vi "IMAG32at.VI"() -> ()   [LabVIEW 2013]
uses:
  Program Files/Andor SOLIS/Drivers 32bit/Examples/LabVIEW/System Files/user.lib/atmcd32d.llb/Shutter_type typedef.ctl
panel:
  out "Intensity Graph":i32[][](graph)
  out "Detector Y Pixels":i32
  in  "Shutter Trigger":T1
  in  "Time to open or\nclose shutter (ms):":i32=50
  in  "Shut Down":bool
  in  "Start Acquisition":bool
  out "Return  from Get Acquired Data":u32
  out "Detector X Pixels":i32
  out "Return from GetStatus":u32
  out "Return from Start Acquisition":u32
  out "Return from CheckTimings Exposure":u32
  out "Calculated Exposure Value":sgl format="%.2f"
  in  "Exposure Time (secs)":sgl=0.05 format="%.2f"
  out "Return from Initialize":u32
  in  "Trigger":u32(ring) items=["Internal", "External"]
  # "Status"
  # "Acquisition Mode: Single Scan\nReadout Mode: Full Resolution\nImage\nOnly show one track of data"
  # "Shutter Trigger"
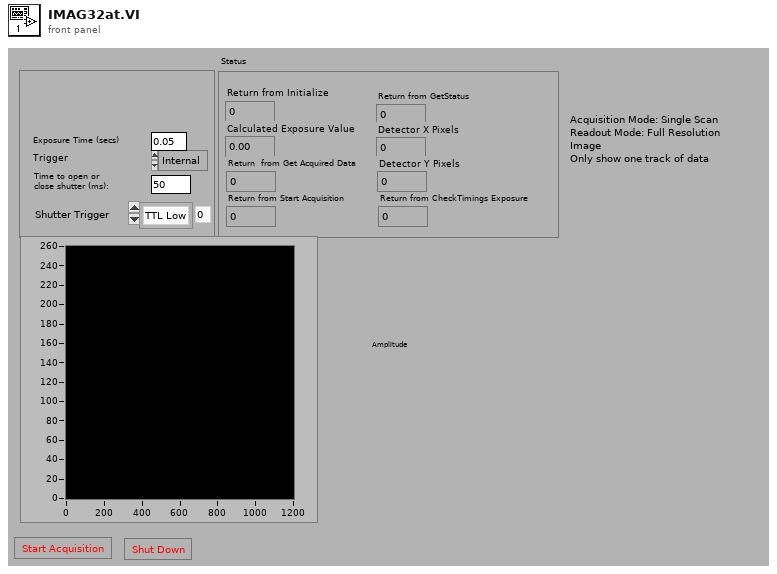
[diagram p1: front panel]
types:
  T1 = typedef "Shutter_type typedef.ctl" = enum16{"TTL Low", "TTL High"}
  T2 = typedef "Error Code Enum typedef.ctl" = enum32{"N/A (0)", "DRV_ERROR_CODES", "DRV_SUCCESS", "DRV_VXDNOTINSTALLED", "DRV_ERROR_SCAN", "DRV_ERROR_CHECK_SUM", "DRV_ERROR_FILELOAD", "DRV_UNKNOWN_FUNC", "DRV_ERROR_VXD_INIT", "DRV_ERROR_ADDRESS", "DRV_ERROR_PAGELOCK", "DRV_ERROR_PAGEUNLOCK", "DRV_ERROR_BOARDTEST", "DRV_ERROR_ACK", "DRV_ERROR_UP_FIFO", "DRV_ERROR_PATTERN", "N/A (16)", "DRV_ACQUISITION_ERRORS", "DRV_ACQ_BUFFER", "DRV_ACQ_DOWNFIFO_FULL", "DRV_PROC_UNKONWN_INSTRUCTION", "DRV_ILLEGAL_OP_CODE", "DRV_KINETIC_TIME_NOT_MET", "DRV_ACCUM_TIME_NOT_MET", "DRV_NO_NEW_DATA", "N/A (25)", "DRV_SPOOLERROR", "N/A (27)", "N/A (28)", "N/A (29)", "N/A (30)", "N/A (31)", "N/A (32)", "DRV_TEMPERATURE_CODES", "DRV_TEMPERATURE_OFF", "DRV_TEMPERATURE_NOT_STABILIZED", "DRV_TEMPERATURE_STABILIZED", "DRV_TEMPERATURE_NOT_REACHED", "DRV_TEMPERATURE_OUT_RANGE", "DRV_TEMPERATURE_NOT_SUPPORTED", "DRV_TEMPERATURE_DRIFT", "N/A (41)", "N/A (42)", "N/A (43)", "N/A (44)", "N/A (45)", "N/A (46)", "N/A (47)", "N/A (48)", "DRV_GENERAL_ERRORS", "DRV_INVALID_AUX", "DRV_COF_NOTLOADED", "DRV_FPGAPROG", "DRV_FLEXERROR", "DRV_GPIBERROR", "N/A (55)", "N/A (56)", "N/A (57)", "N/A (58)", "N/A (59)", "N/A (60)", "N/A (61)", "N/A (62)", "N/A (63)", "DRV_DATATYPE", "DRV_DRIVER_ERRORS", "DRV_P1INVALID", "DRV_P2INVALID", "DRV_P3INVALID", "DRV_P4INVALID", "DRV_INIERROR", "DRV_COFERROR", "DRV_ACQUIRING", "DRV_IDLE", "DRV_TEMPCYCLE", "DRV_NOT_INITIALIZED", "DRV_P5INVALID", "DRV_P6INVALID", "DRV_INVALID_MODE", "DRV_INVALID_FILTER", "DRV_I2CERRORS", "DRV_I2CDEVNOTFOUND", "DRV_I2CTIMEOUT", "DRV_P7INVALID", "N/A (84)", "N/A (85)", "N/A (86)", "N/A (87)", "N/A (88)", "N/A (89)", "DRV_IOCERROR", "DRV_VRMVERSIONERROR"}
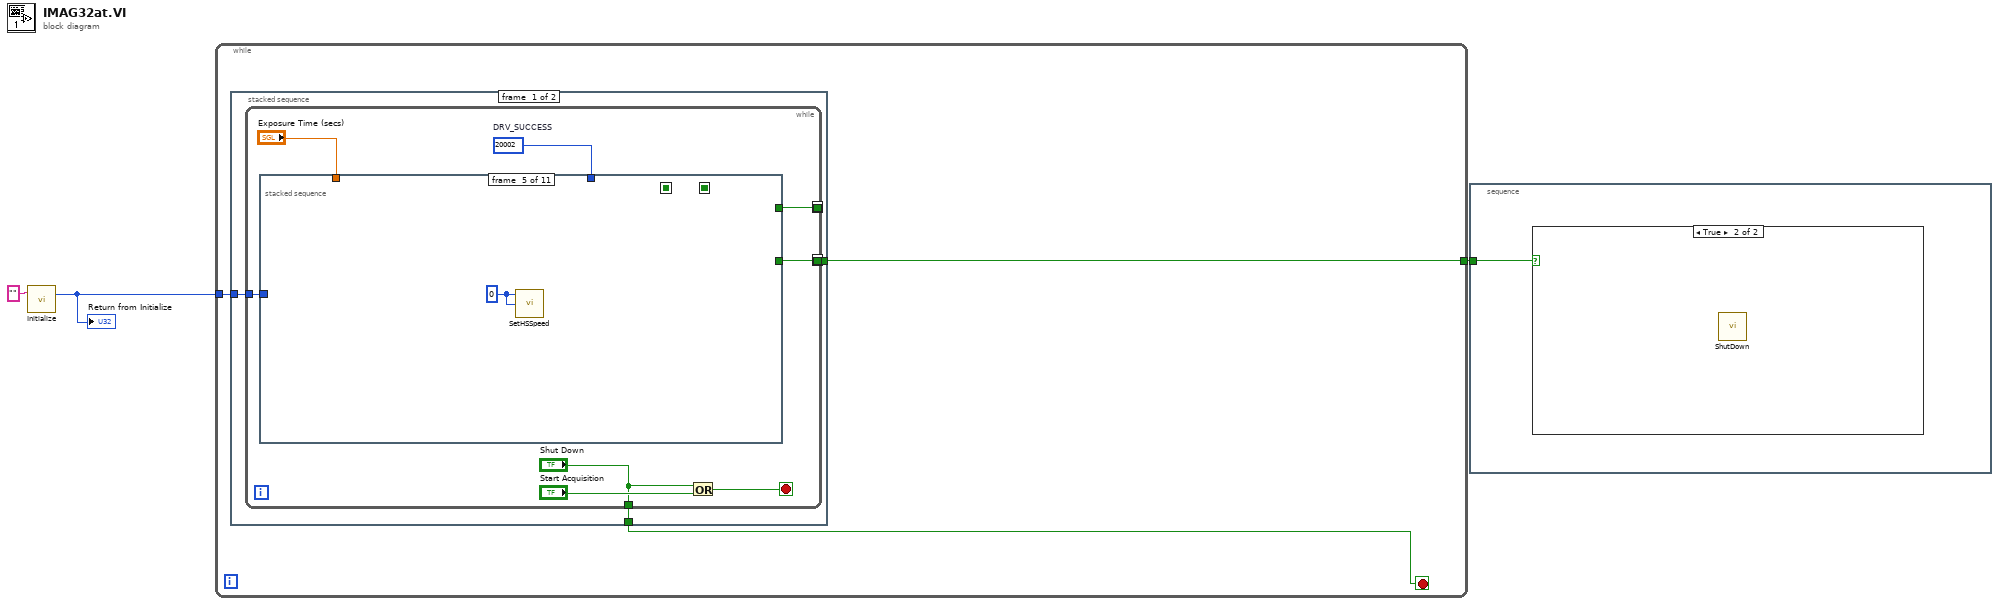
[diagram p0: block diagram]
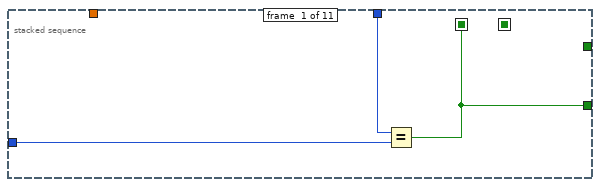
[diagram p2: hidden frame]
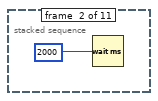
[diagram p3: hidden frame]
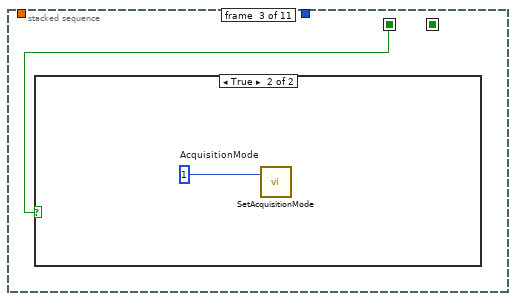
[diagram p4: hidden frame]
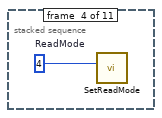
[diagram p6: hidden frame]
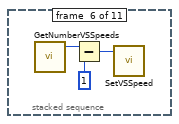
[diagram p7: hidden frame]
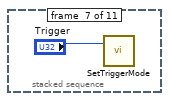
[diagram p8: hidden frame]
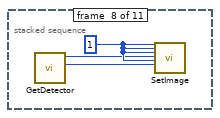
[diagram p9: hidden frame]
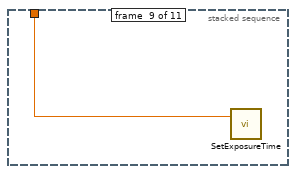
[diagram p10: hidden frame]
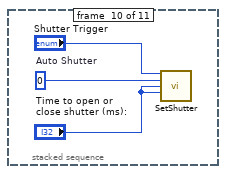
[diagram p11: hidden frame]
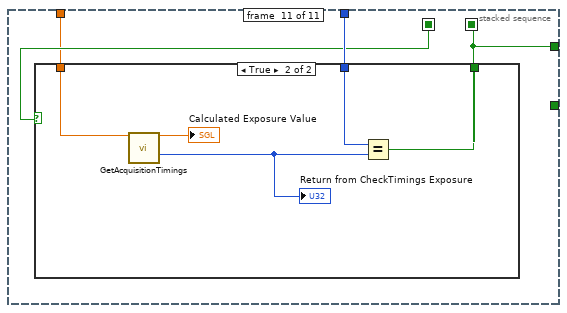
[diagram p12: hidden frame]
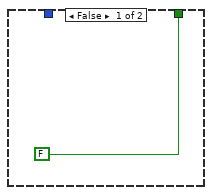
[diagram p13: hidden frame]
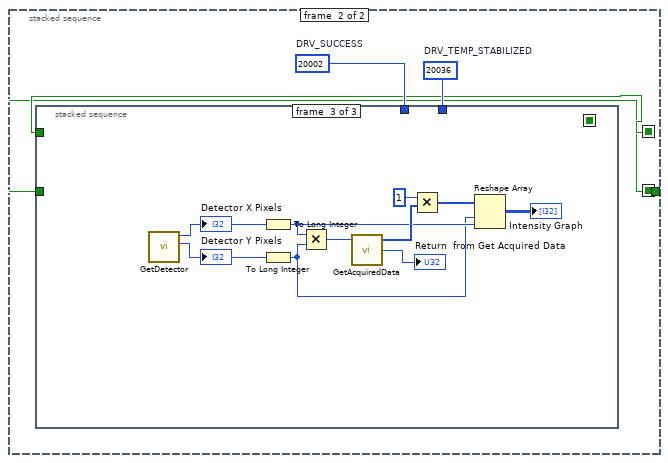
[diagram p14: hidden frame]
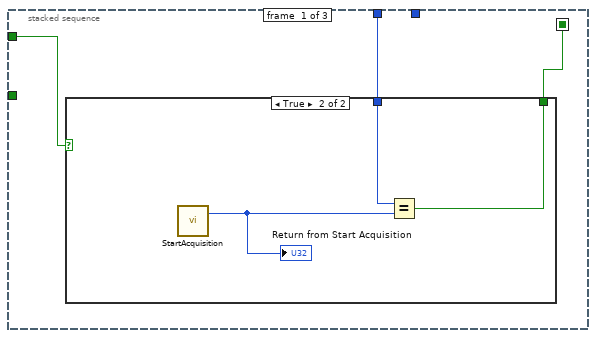
[diagram p15: hidden frame]
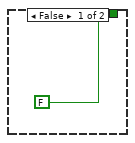
[diagram p16: hidden frame]
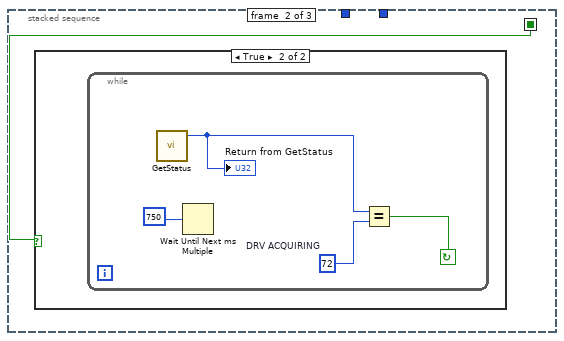
[diagram p17: hidden frame]
diagram:
  n1 = call "Initialize.vi"("directory (\"\")"="" ("directory (\"\")")) -> ("DLL error code"=w2:u32)  [unwired: 1 in, 1 out]
  "Return from Initialize" <- w2
  n2 = while {
    tunnel: w2 -> [w6]
    tunnel: [w5] -> w1
    stop <- w4 stop-if-true
    n3 = stacked-sequence {
      seq-local: [w9 _] -> [_ w49]
      seq-local: [w8 _] -> [_ w48]
      tunnel: w6 -> [w10 _]
      tunnel: [w7 _] -> w4
      tunnel: [_ w48] -> w5
      frame #0 {
        n4 = while {
          tunnel: w10 -> [w16]
          tunnel: [w15] -> w9
          tunnel: [w14] -> w8
          tunnel: ["Shut Down"] -> w7
          stop <- w12 stop-if-true
          w17 = 20002  # DRV_SUCCESS
          n5 = stacked-sequence {
            seq-local: [w19 _ _ _ _ _ _ _ _ _ _] -> [_ _ w23 _ _ _ _ _ _ _ w40]
            seq-local: [_ _ _ _ _ _ _ _ _ _ w38] -> [_ _ _ _ _ _ _ _ _ _ _]
            tunnel: "Exposure Time (secs)" -> [_ _ _ _ _ _ _ _ w34 _ w39]
            tunnel: w17 -> [w21 _ _ _ _ _ _ _ _ _ w41]
            tunnel: w16 -> [w20 _ _ _ _ _ _ _ _ _ _]
            tunnel: [_ _ _ _ _ _ _ _ _ _ w38] -> w15
            tunnel: [w19 _ _ _ _ _ _ _ _ _ _] -> w14
            frame #0 {
              n6 = Equal?(x=w21, y=w20) -> (x = y?=w19:bool)
            }
            frame #1 {
              n7 = Wait (ms)(milliseconds to wait=u32 2000) -> ()  [unwired: 1 out]
            }
            frame #2 {
              n8 = case shown="True" w23 {
                frame False {
                }
                frame True {
                  w24 = u16 1  # AcquisitionMode
                  n9 = call "SetAcquisitionMode.vi"("mode"=w24) -> ()  [unwired: 1 in, 2 out]
                }
              }
            }
            frame #3 {
              w25 = u16 4  # ReadMode
              n10 = call "SetReadMode.vi"("mode"=w25) -> ()  [unwired: 1 in, 2 out]
            }
            frame #4 {
              w26 = 0
              n11 = call "SetHSSpeed.vi"("index"=w26, "type"=w26) -> ()  [unwired: 2 in, 2 out]
            }
            frame #5 {
              n12 = call "GetNumberVSSpeeds.vi"() -> ("number"=w29:i32)  [unwired: 3 in, 2 out]
              n13 = Subtract(x=w29, y=1) -> (x-y=w27:i32)
              n14 = call "SetVSSpeed.vi"("index"=w27) -> ()  [unwired: 1 in, 2 out]
            }
            frame #6 {
              n15 = call "SetTriggerMode.vi"("mode"="Trigger") -> ()  [unwired: 1 in, 2 out]
            }
            frame #7 {
              w33 = 1 ("hbin")
              n16 = call "GetDetector.vi"() -> ("ypixels"=w31:i32, "xpixels"=w32:i32)  [unwired: 4 in, 2 out]
              n17 = call "SetImage.vi"("hbin"=w33, "vbin"=w33, "hstart"=w33, "hend"=w32, "vstart"=w33, "vend"=w31) -> ()  [unwired: 20 in, 2 out]
            }
            frame #8 {
              n18 = call "SetExposureTime.vi"("time"=w34) -> ()  [unwired: 1 in, 2 out]
            }
            frame #9 {
              w36 = 0  # Auto Shutter
              n19 = call "SetShutter.vi"("type"="Shutter Trigger", "mode"=w36, "closingtime"="Time to open or\nclose shutter (ms):", "openingtime"="Time to open or\nclose shutter (ms):") -> ()  [unwired: 10 in, 2 out]
            }
            frame #10 {
              n20 = case shown="True" w40 {
                tunnel: w41 -> [_ w44]
                tunnel: [FALSE w47] -> w38
                tunnel: w39 -> [_ w45]
                frame False {
                }
                frame True {
                  n21 = call "GetAcquisitionTimings.vi"("exposure input"=w45) -> ("exposure"=→"Calculated Exposure Value":sgl, "DLL error code"=w43:u32)  [unwired: 10 in, 3 out]
                  "Return from CheckTimings Exposure" <- w43
                  n22 = Equal?(x=w44, y=w43) -> (x = y?=w47:bool)
                }
              }
            }
          }
          n23 = Or(x="Shut Down", y="Start Acquisition") -> (x .or. y?=w12:bool)
        }
      }
      frame #1 {
        w50 = 20036  # DRV_TEMP_STABILIZED
        w51 = 20002  # DRV_SUCCESS
        n24 = stacked-sequence {
          seq-local: [w53 _ _] -> [_ w59 _]
          tunnel: w51 -> [w54 _ _]
          tunnel: w50 -> [_ _ _]
          tunnel: w49 -> [w52 _ _]
          tunnel: w48 -> [_ _ _]
          frame #0 {
            n25 = case shown="True" w52 {
              tunnel: [FALSE w58] -> w53
              tunnel: w54 -> [_ w57]
              frame False {
              }
              frame True {
                n26 = call "StartAcquisition.vi"() -> ("DLL error code"=w56:u32)  [unwired: 2 in, 1 out]
                "Return from Start Acquisition" <- w56
                n27 = Equal?(x=w57, y=w56) -> (x = y?=w58:bool)
              }
            }
          }
          frame #1 {
            n28 = case shown="True" w59 {
              frame False {
              }
              frame True {
                n29 = while {
                  stop <- w62 continue-if-true
                  w61 = u16 72  # DRV ACQUIRING
                  n30 = call "GetStatus.vi"() -> ("status"=w60:T2)  [unwired: 3 in, 2 out]
                  "Return from GetStatus" <- w60
                  n31 = Wait Until Next ms Multiple(millisecond multiple=u32 750) -> ()  [unwired: 1 out]
                  n32 = Equal?(x=w60, y=w61) -> (x = y?=w62:bool)
                }
              }
            }
          }
          frame #2 {
            n33 = call "GetDetector.vi"() -> ("ypixels"=w70:i32, "xpixels"=w73:i32)  [unwired: 4 in, 2 out]
            "Detector X Pixels" <- w73
            "Detector Y Pixels" <- w70
            n34 = To Long Integer(number=w73) -> (32bit integer=w65:i32)
            n35 = To Long Integer(number=w70) -> (32bit integer=w64:i32)
            n36 = Multiply(x=w65, y=w64) -> (x*y=w71:i32)
            n37 = call "GetAcquiredData.vi"("size"=w71) -> ("DLL error code"=→"Return  from Get Acquired Data":u32, "array"=w68:i32[])  [unwired: 2 in, 1 out]
            n38 = Multiply(x=1, y=w68) -> (x*y=w67:i32[])
            n39 = Reshape Array(w67, w64, w65) -> (→"Intensity Graph":i32[][])
          }
        }
      }
    }
  }
  n40 = stacked-sequence {
    tunnel: w1 -> [w74]
    frame #0 {
      n41 = case shown="True" w74 {
        frame False {
        }
        frame True {
          n42 = call "ShutDown.vi"() -> ()  [unwired: 2 in, 2 out]
        }
      }
    }
  }
